vi "窗位窗宽调整子VI.vi"(7 "Image in":T1, 8 "Palette:User Palette":cluster{"Red":u8, "Green":u8, "Blue":u8}[](array[cluster]), 9 "Palette:Palette Type":u32(ring) items=["Grayscale", "Binary", "Gradient", "Rainbow", "Temperature", "User Defined", "Binary 16 Bit", "Gradient 16 Bit", "Rainbow 16 Bit", "Temperature 16 Bit", "User Defined 16 Bit"], 11 "Image Pixels (U8)":u8[][](array[numeric])) -> (3 "Image out":T1(plugin-control))   [LabVIEW 2018]
uses:
  <vilib>/vision/Image Controls.llb/IMAQ Image.ctl
  <vilib>/vision/NI_Vision_Development_Module.lvlib
panel:
  in  "阈值范围选择":cluster{u8, u8}(slide)={50, 212} scale=0.0..255.0
  in  "确定":bool
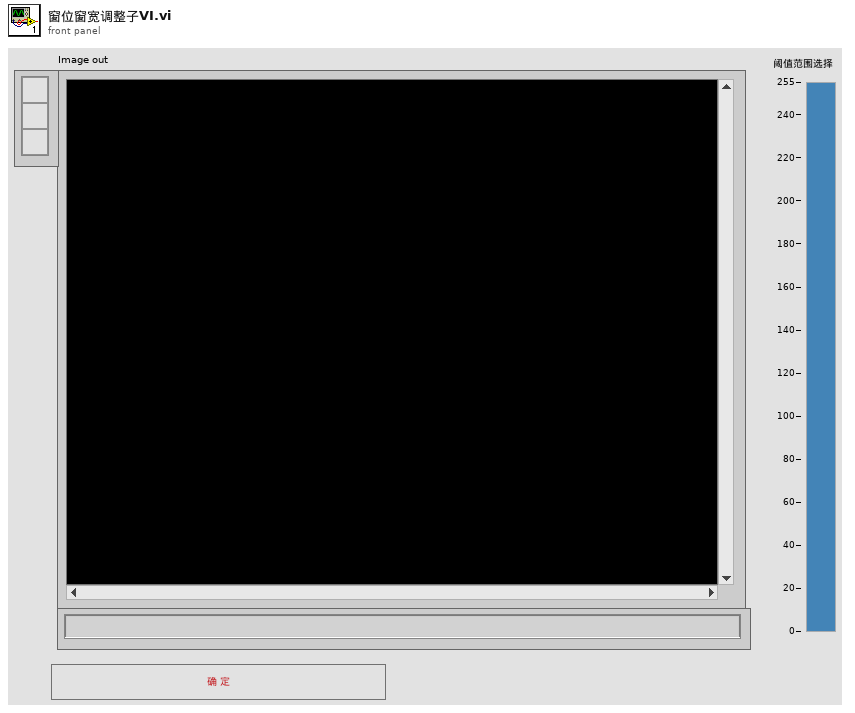
[diagram p1: front panel]
types:
  T1 = typedef "IMAQ Image.ctl" = refnum<image>
  T2 = cluster{"Zoom Tool":bool, "Selection Tool":bool, "Pan Tool":bool, "Point Tool":bool, "Line Tool":bool, "Rectangle Tool":bool, "Rotated Rectangle Tool":bool, "Polyline Tool":bool, "Polygon Tool":bool, "Freehand Tool":bool, "Closed Freehand Tool":bool, "Ellipse Tool":bool, "Annulus Tool":bool}
  T3 = enum32{"Linear", "Log", "Exp", "Square", "Square root", "Power X", "Power 1/X"}
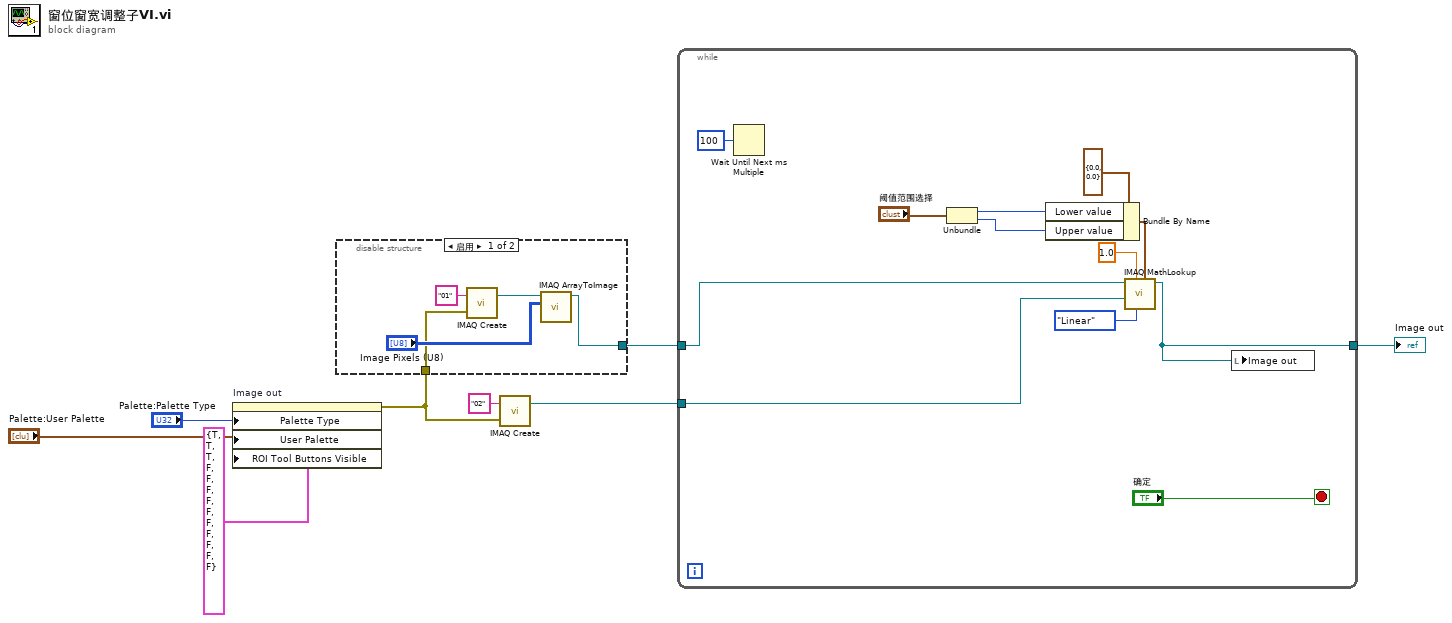
[diagram p0: block diagram]
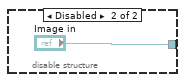
[diagram p2: hidden frame]
diagram:
  n1 = property on="Image out" class="ImageControl"("Palette Type"="Palette:Palette Type", "User Palette"="Palette:User Palette", "ROI Tool Buttons Visible"=T2 {"Zoom Tool"=TRUE, "Selection Tool"=TRUE, "Pan Tool"=TRUE, "Point Tool"=FALSE, "Line Tool"=FALSE, "Rectangle Tool"=FALSE, "Rotated Rectangle Tool"=FALSE, "Polyline Tool"=FALSE, "Polygon Tool"=FALSE, "Freehand Tool"=FALSE, "Closed Freehand Tool"=FALSE, "Ellipse Tool"=FALSE, "Annulus Tool"=FALSE} ("ROI Tool Buttons Visible:All Elements")) -> (error out=w3:errorcluster)  [unwired: 2 in, 1 out]
  n2 = disable-structure shown="启用" {
    disable-tunnel: [w10 "Image in"] -> w4
    disable-tunnel: w3 -> [w9 _]
    frame Enabled {
      n3 = call "IMAQ Create"("Image Name"="01", "error in (no error)"=w9) -> ("New Image"=w12:T1)  [unwired: 3 in, 1 out]
      n4 = call "IMAQ ArrayToImage"("Image Pixels (U8)"="Image Pixels (U8)", "Image"=w12) -> ("Image Out"=w10:T1)  [unwired: 8 in, 1 out]
    }
    frame Disabled {
    }
  }
  n5 = call "IMAQ Create"("Image Name"="02", "error in (no error)"=w3) -> ("New Image"=w8:T1)  [unwired: 3 in, 1 out]
  n6 = while {
    tunnel: w8 -> [w15]
    tunnel: w4 -> [w17]
    tunnel: [w16] -> w1
    stop <- "确定" stop-if-true
    n7 = Wait Until Next ms Multiple(millisecond multiple=u32 100 ("毫秒倍数")) -> ()  [unwired: 1 out]
    n8 = Unbundle("阈值范围选择") -> (w24:u8, w23:u8)
    n9 = Bundle By Name(cluster=cluster{"Lower value":sgl, "Upper value":sgl} {"Lower value"=0.0, "Upper value"=0.0} ("输入簇"), "Lower value"=w24, "Upper value"=w23) -> (w22:cluster{"Lower value":sgl, "Upper value":sgl})
    n10 = call "IMAQ MathLookup"("Range"=w22, "Operator"=T3."Linear", "X Value"=sgl 1.0, "Image Dst"=w15, "Image Src"=w17) -> ("Image Dst Out"=w16:T1)  [unwired: 5 in, 1 out]
    n11 = local write "Image out"(w16) -> ()
  }
  "Image out" <- w1
